vi "GetParamAndUnitFromCommand.vi"(11 "SetParameter":T1) -> (2 "Parameter":string, 3 "Unit Label":string)   [LabVIEW 2018]
uses:
  TypeDefs/SetParameterInputs.ctl
  AcPwrBase.lvclass
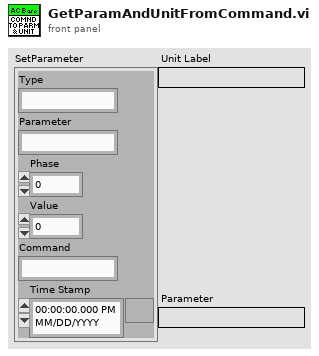
[diagram p1: front panel]
types:
  T1 = typedef "AcPwrPlugins.lvlib/AcPwrBase.lvclass/SetParameterInputs.ctl" = cluster{"Type":string, "Parameter":string, "Phase":i32, "Value":dbl, "Command":string, "Time Stamp":timestamp}
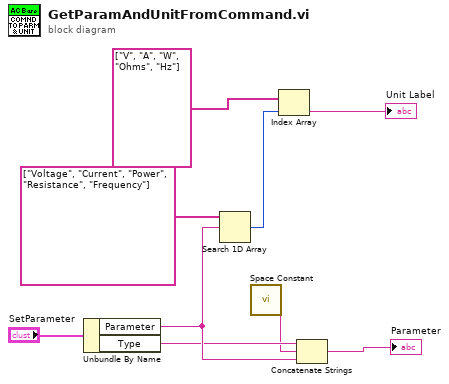
[diagram p0: block diagram]
diagram:
  n1 = Unbundle By Name("SetParameter") -> ("Parameter"=w4:string, "Type"=w2:string)
  n2 = Search 1D Array(1D array=string[] ["Voltage", "Current", "Power", "Resistance", "Frequency"] ("Handle"), element=w4) -> (index of element=w5:i32)  [unwired: 1 in]
  n3 = call <vilib>:"Space Constant.vi"() -> ("String"=w1:string)
  n4 = Index Array(array=string[] ["V", "A", "W", "Ohms", "Hz"] ("Handle"), index=w5) -> (element=→"Unit Label":string)
  n5 = Concatenate Strings(w2, w1, w4) -> (→"Parameter":string)
